vi "State Machine_Pretzel Dispenser.vi"() -> ()   [LabVIEW 2020]
panel:
  out "$ Charged":dbl
  out "Dispense\nChange":bool
  out "Change\nDispensed ($)":dbl format="%.2f"
  out "Vend":bool
  out "Money\nInserted ($)":dbl format="%.2g"
  in  "Payment Type":T1(ring)
  in  "Insert Payment":bool
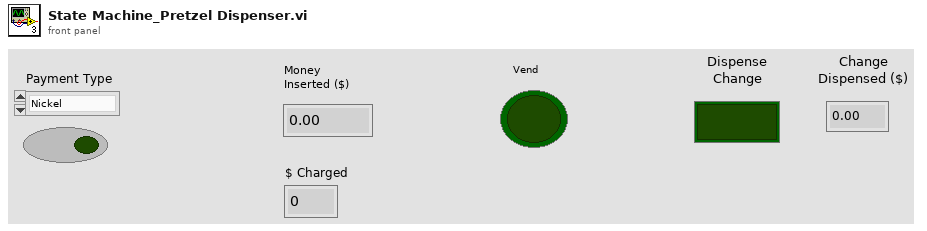
[diagram p1: front panel]
types:
  T1 = enum16{"Nickel", "Dime", "Quarter", "Card Swipe", "Shutdown", "Vend", "Change", "Wait", "Initialize"}
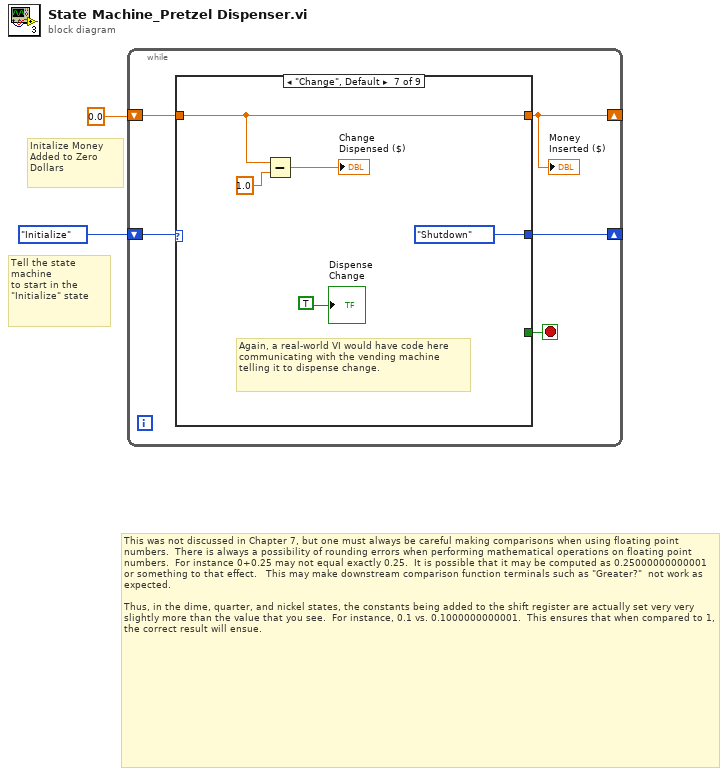
[diagram p0: block diagram]
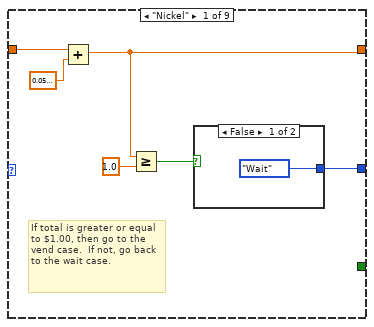
[diagram p2: hidden frame]
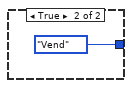
[diagram p3: hidden frame]
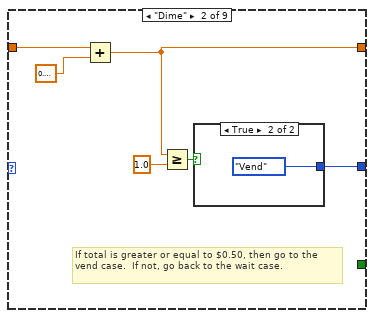
[diagram p4: hidden frame]
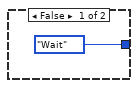
[diagram p5: hidden frame]
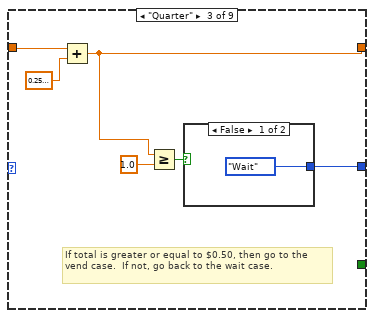
[diagram p6: hidden frame]
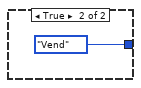
[diagram p7: hidden frame]
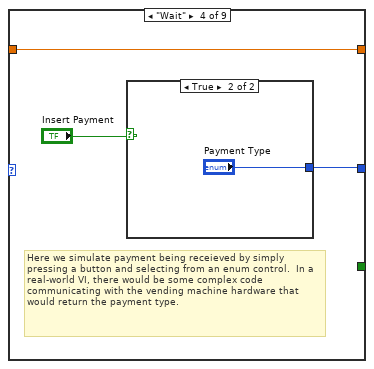
[diagram p8: hidden frame]
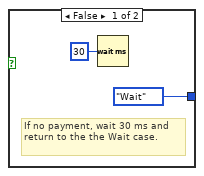
[diagram p9: hidden frame]
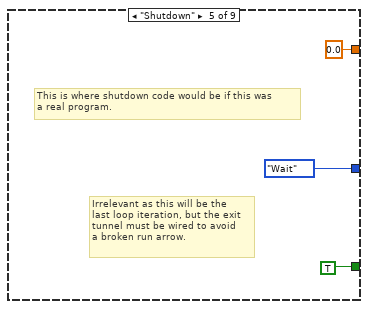
[diagram p10: hidden frame]
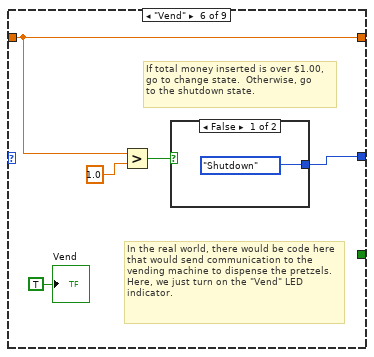
[diagram p11: hidden frame]
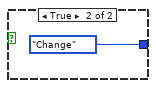
[diagram p12: hidden frame]
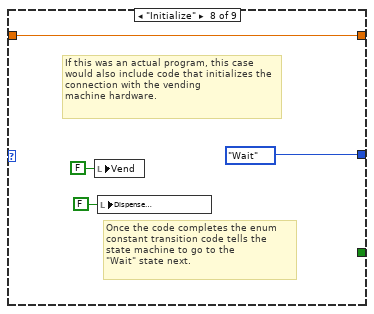
[diagram p13: hidden frame]
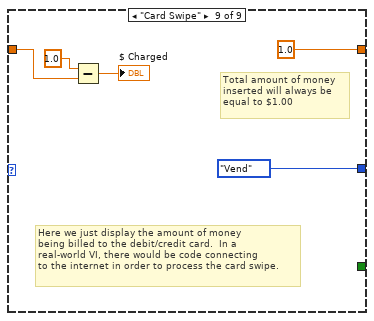
[diagram p14: hidden frame]
diagram:
  # "This was not discussed in Chapter 7, but one must always be careful making comparisons when using floating point numbers.  There is always a possibility of rounding errors when performing mathematical operations on floating point numbers.  For instance 0+0.25 may not equal exactly 0.25.  It is possible that it may be computed as 0.25000000000001 or something to that effect.   This may make downstream comparison function terminals such as \"Greater?\"  not work as expected.\n\nThus, in the dime, quarter, and nickel states, the constants being added to the shift register are actually set very very slightly more than the value that you see.  For instance, 0.1 vs. 0.1000000000001.  This ensures that when compared to 1, the correct result will ensue."
  # "Tell the state machine\nto start in the \"Initialize\" state"
  # "Initalize Money\nAdded to Zero Dollars"
  n1 = while {
    shift-right: [w6] -> _
    shift-left: T1."Initialize" ("Payment Type") -> [w7]
    shift-right: [w4] -> _
    shift-left: 0.0 -> [w5]
    stop <- w3 stop-if-true
    n2 = case shown="\"Change\", Default" w7 {
      tunnel: [w13 w21 w29 w33 T1."Wait" ("Payment Type") w45 T1."Shutdown" ("Payment Type") T1."Wait" ("Payment Type") T1."Vend" ("Payment Type")] -> w6
      tunnel: w5 -> [w12 w20 w28 w32 _ w41 w52 w56 w59]
      tunnel: [w9 w17 w26 w32 0.0 w41 w52 w56 1.0] -> w4
      tunnel: [_ _ _ _ TRUE _ _ _ _] -> w3
      frame "Nickel" {
        # "If total is greater or equal to $1.00, then go to the vend case.  If not, go back to the wait case."
        n3 = Add(x=w12, y=0.0500000000001) -> (x+y=w9:dbl)
        n4 = Greater Or Equal?(x=w9, y=1.0) -> (x >= y?=w10:bool)
        n5 = case shown="False" w10 {
          tunnel: [T1."Wait" ("Payment Type") T1."Vend" ("Payment Type")] -> w13
          frame False {
          }
          frame True {
          }
        }
      }
      frame "Dime" {
        # "If total is greater or equal to $0.50, then go to the vend case.  If not, go back to the wait case."
        n6 = Add(x=w20, y=0.1000000000001) -> (x+y=w17:dbl)
        n7 = Greater Or Equal?(x=w17, y=1.0) -> (x >= y?=w18:bool)
        n8 = case shown="True" w18 {
          tunnel: [T1."Wait" ("Payment Type") T1."Vend" ("Payment Type")] -> w21
          frame False {
          }
          frame True {
          }
        }
      }
      frame "Quarter" {
        # "If total is greater or equal to $0.50, then go to the vend case.  If not, go back to the wait case."
        n9 = Add(x=w28, y=0.2500000000000001) -> (x+y=w26:dbl)
        n10 = Greater Or Equal?(x=w26, y=1.0) -> (x >= y?=w27:bool)
        n11 = case shown="False" w27 {
          tunnel: [T1."Wait" ("Payment Type") T1."Vend" ("Payment Type")] -> w29
          frame False {
          }
          frame True {
          }
        }
      }
      frame "Wait" {
        # "Here we simulate payment being receieved by simply pressing a button and selecting from an enum control.  In a real-world VI, there would be some complex code communicating with the vending machine hardware that would return the payment type."
        n12 = case shown="True" "Insert Payment" {
          tunnel: [T1."Wait" ("Payment Type") "Payment Type"] -> w33
          frame False {
            # "If no payment, wait 30 ms and return to the the Wait case."
            n13 = Wait (ms)(milliseconds to wait=u32 30) -> ()  [unwired: 1 out]
          }
          frame True {
          }
        }
      }
      frame "Shutdown" {
        # "Irrelevant as this will be the \nlast loop iteration, but the exit\ntunnel must be wired to avoid \na broken run arrow."
        # "This is where shutdown code would be if this was \na real program."
      }
      frame "Vend" {
        # "In the real world, there would be code here that would send communication to the vending machine to dispense the pretzels.  Here, we just turn on the \"Vend\" LED indicator."
        # "If total money inserted is over $1.00,\ngo to change state.  Otherwise, go\nto the shutdown state."
        n14 = Greater?(x=w41, y=1.0) -> (0:w43:bool)
        n15 = case shown="False" w43 {
          tunnel: [T1."Shutdown" ("Payment Type") T1."Change" ("Payment Type")] -> w45
          frame False {
          }
          frame True {
          }
        }
        "Vend" <- TRUE ("Vend Soda")
      }
      frame "Change", Default {
        # "Again, a real-world VI would have code here communicating with the vending machine telling it to dispense change."
        n16 = Subtract(x=w52, y=1.0) -> (x-y=→"Change\nDispensed ($)":dbl)
        "Dispense\nChange" <- TRUE ("Dispense\nChange")
      }
      frame "Initialize" {
        # "Once the code completes the enum constant transition code tells the state machine to go to the \n\"Wait\" state next."
        # "If this was an actual program, this case would also include code that initializes the connection with the vending\nmachine hardware."
        n17 = local write "Vend"(FALSE ("Vend")) -> ()
        n18 = local write "Dispense\nChange"(FALSE ("Dispense\nChange")) -> ()
      }
      frame "Card Swipe" {
        # "Here we just display the amount of money\nbeing billed to the debit/credit card.  In a \nreal-world VI, there would be code connecting\nto the internet in order to process the card swipe."
        # "Total amount of money\ninserted will always be\nequal to $1.00"
        n19 = Subtract(x=1.0, y=w59) -> (x-y=→"$ Charged":dbl)
      }
    }
    "Money\nInserted ($)" <- w4
  }
